vi "SRV_Initialize Motor Buttons.vi"(0 "Motors Config File Path":path, 1 "button refs":refnum<vi>[](array[refnum]), 5 "false refs":refnum<vi>[](array[refnum]), 7 "true refs":refnum<vi>[](array[refnum]), 9 "Init from File (F)":bool, 11 "error in (no error)":errorcluster) -> (8 "Motor Control Config":T1[](array[typedef]) {"Release Cmds"."Motor Control Commands Array"."Value" format="%02x"; "Release Cmds"."Motor Control Commands Array"."Register" format="%02x"; "Release Cmds"."Motor Control Commands Array"."I2C Address" format="%02x"; "Press Cmds"."Motor Control Commands Array"."Value" format="%02x"; "Press Cmds"."Motor Control Commands Array"."Register" format="%02x"; "Press Cmds"."Motor Control Commands Array"."I2C Address" format="%02x"}, 15 "error out":errorcluster)   [LabVIEW 2014]
doc: "Author: Mike Schultz (LogicPD, Inc)"
uses:
  Motors Config/SRV_Motor Control Button Config.ctl
  Motors Config/SRV_Motor Legos-Servo.ctl
  Motors Config/SRV_Motor Control Commands Cluster.ctl
  Motors Config/SRV_Motor Control Command Config.ctl
  Motors Config/SRV_Motor Control Button Icons_FALSE.ctl
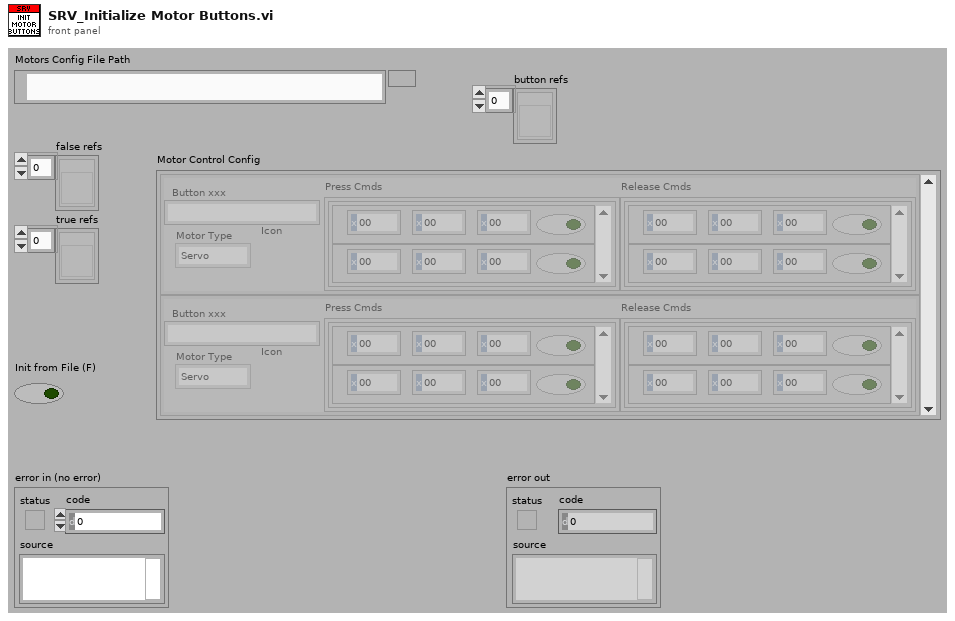
[diagram p1: front panel]
types:
  T1 = typedef "SRV_Motor Control Button Config.ctl" = cluster{"Button Name":string, "Button Label":string, "Motor Type":T2, "Press Cmds":T3, "Release Cmds":T3, "Icon":T5}
  T2 = typedef "SRV_Motor Legos-Servo.ctl" = enum16{"Servo", "Legos", "Shared Var"}
  T3 = typedef "SRV_Motor Control Commands Cluster.ctl" = cluster{"Motor Control Commands Array":T4[]}
  T4 = typedef "SRV_Motor Control Command Config.ctl" = cluster{"I2C Address":u8, "Register":u8, "Value":u8, "Active":bool}
  T5 = typedef "SRV_Motor Control Button Icons_FALSE.ctl" = u16
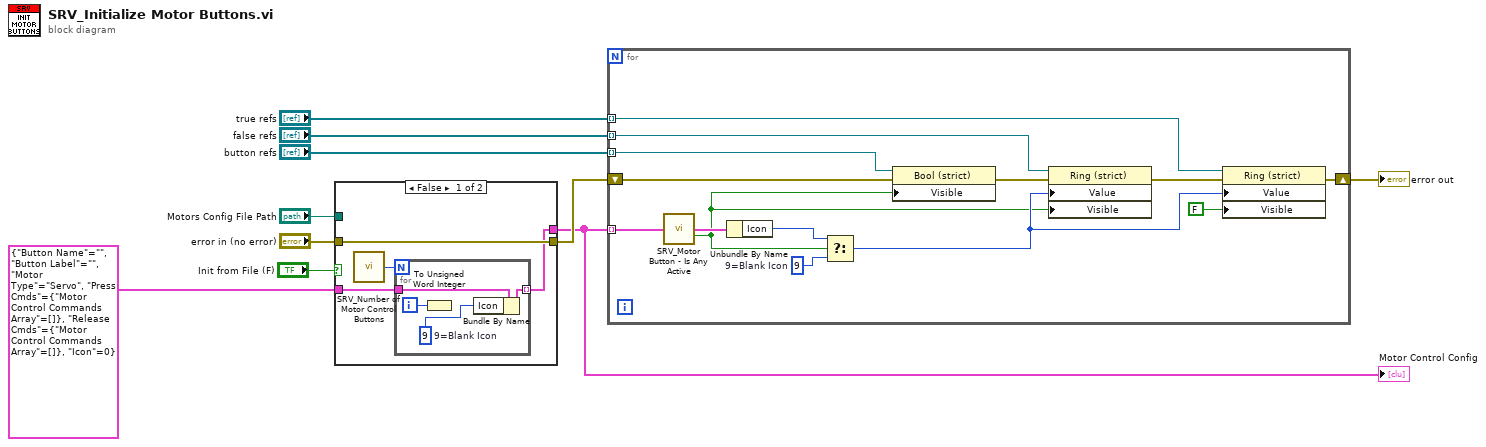
[diagram p0: block diagram]
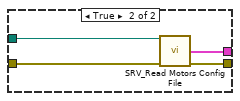
[diagram p2: hidden frame]
diagram:
  n1 = case shown="False" "Init from File (F)" {
    tunnel: "error in (no error)" -> [w14 w22]
    tunnel: "Motors Config File Path" -> [_ w21]
    tunnel: [w14 w20] -> w7
    tunnel: [w12 w19] -> w4
    tunnel: T1 {"Button Name"="", "Button Label"="", "Motor Type"=enum."Servo", "Press Cmds"={"Motor Control Commands Array"=[]}, "Release Cmds"={"Motor Control Commands Array"=[]}, "Icon"=0} ("Motor Control Button") -> [w13 _]
    frame False {
      n2 = call "SRV_Number of Motor Control Buttons.vi"() -> ("Number of Motor Control Buttons"=w11:i32)  [unwired: 14 in, 1 out]
      n3 = for {
        N: w11 -> [_]
        tunnel: w13 -> [w18]
        tunnel: [w17] -> w12 mode=indexing
        i -> [w16]
        w15 = T5 9  # 9=Blank Icon
        n4 = To Unsigned Word Integer(number=w16) -> ()  [unwired: 1 out]
        n5 = Bundle By Name(cluster=w18, "Icon"=w15) -> (w17:T1)
      }
    }
    frame True {
      n6 = call "SRV_Read Motors Config File.vi"("Motors Config File Path"=w21, "error in (no error)"=w22) -> ("Motor Control Config"=w19:T1[], "error out"=w20:errorcluster)  [unwired: 10 in, 2 out]
    }
  }
  "Motor Control Config" <- w4
  n7 = for {
    tunnel: w4 -> [w32] mode=indexing
    tunnel: "false refs" -> [w36] mode=indexing
    shift-right: [w34] -> w5
    shift-left: w7 -> [w26]
    tunnel: "true refs" -> [w35] mode=indexing
    tunnel: "button refs" -> [w24] mode=indexing
    w28 = T5 9  # 9=Blank Icon
    n8 = call "SRV_Motor Button - Is Any Active.vi"("Motor Control Button"=w32) -> ("Motor Control Button dup"=w31:T1, "Any Active?"=w23:bool)  [unwired: 13 in]
    n9 = Unbundle By Name(w31) -> ("Icon"=w30:T5)
    n10 = Select(t=w30, s=w23, f=w28) -> (s? t:f=w29:T5)
    n11 = property class="Bool (strict)"(reference=w24, error in=w26, "Visible"=w23) -> (error out=w25:errorcluster)  [unwired: 1 out]
    n12 = property class="Ring (strict)"(reference=w36, error in=w25, "Value"=w29, "Visible"=w23) -> (error out=w27:errorcluster)  [unwired: 1 out]
    n13 = property class="Ring (strict)"(reference=w35, error in=w27, "Value"=w29, "Visible"=FALSE) -> (error out=w34:errorcluster)  [unwired: 1 out]
  }
  "error out" <- w5
